vi "DSF.Engine.Memory.Cache.Plugin.Get Transfer Group Cache.vi"(10 "Transfer Group ID":i32, 11 "Plugin Cache in":refnum<class "DSF.Engine.Memory.Cache.Plugin.lvclass">) -> (2 "Transfer Group Cache":refnum<class "DSF.Engine.Memory.Cache.Transfer Group.lvclass">, 3 "Plugin Cache out":refnum<class "DSF.Engine.Memory.Cache.Plugin.lvclass">)   [LabVIEW 2016, in "DSF.Engine.lvlib" / "DSF.Engine.Memory.Cache.Plugin.lvclass"]
uses:
  DSF.Engine.Memory.Cache.Plugin.lvclass
  DSF.Engine.Memory.Cache.Transfer Group.lvclass
  DSF.Engine.Memory.Cache.Plugin.lvclass/DSF.Engine.Memory.Cache.Plugin.ctl
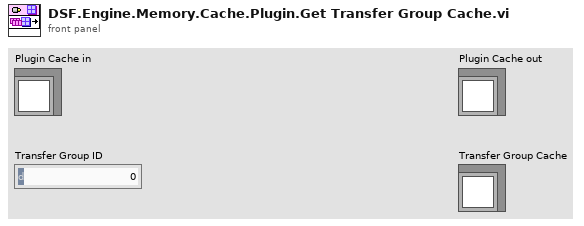
[diagram p1: front panel]
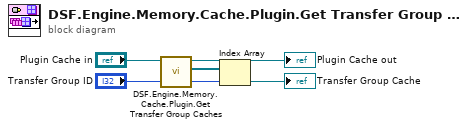
[diagram p0: block diagram]
diagram:
  n1 = call "DSF.Engine.Memory.Cache.Plugin.Get Transfer Group Caches.vi"("Plugin Cache in"="Plugin Cache in") -> ("Transfer Group Caches"=w3:refnum<class "DSF.Engine.Memory.Cache.Transfer Group.lvclass">[], "Plugin Cache out"=→"Plugin Cache out":refnum<class "DSF.Engine.Memory.Cache.Plugin.lvclass">)  [unwired: 9 in]
  n2 = Index Array(array=w3, index="Transfer Group ID") -> (element=→"Transfer Group Cache":refnum<class "DSF.Engine.Memory.Cache.Transfer Group.lvclass">)
